vi "CreateProduct.vi"(8 "error in (no error)":errorcluster, 11 "Factory in":refnum<class "Factory.lvclass">) -> (0 "error out":errorcluster, 2 "Product.lvclass":refnum<class "Product.lvclass">, 3 "Factory out":refnum<class "Factory.lvclass">)   [LabVIEW 2018, in "Factory.lvclass"]
uses:
  Factory.lvclass
  Product Class/Product/Product.lvclass
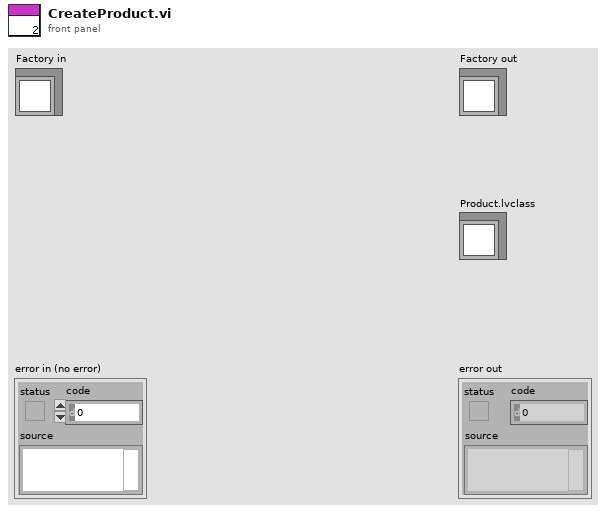
[diagram p1: front panel]
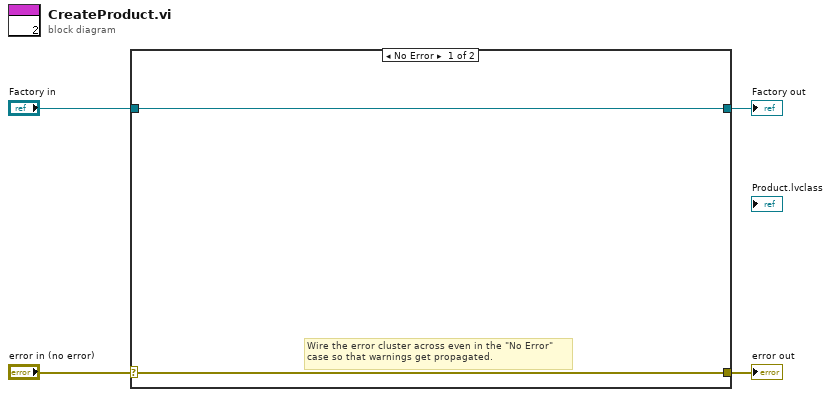
[diagram p0: block diagram]
diagram:
  n1 = case shown="No Error" "error in (no error)" {
    selector: "error in (no error)" -> [w5 w8]
    tunnel: [w5 w8] -> w3
    tunnel: [w6 w7] -> w1
    tunnel: "Factory in" -> [w6 w7]
    frame No Error {
      # "Wire the error cluster across even in the \"No Error\"\ncase so that warnings get propagated."
    }
    frame Error {
    }
  }
  "error out" <- w3
  "Factory out" <- w1
